vi "0-999 NUMBER TO STRING (SubVI).vi"(1 "A":dbl) -> (0 "element":string)   [LabVIEW 2019]
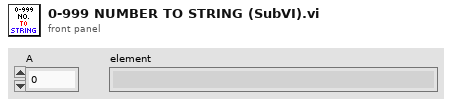
[diagram p1: front panel]
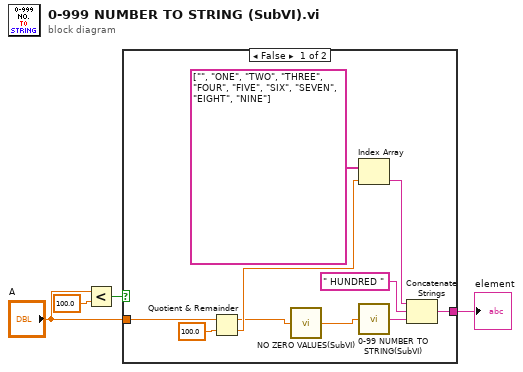
[diagram p0: block diagram]
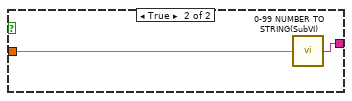
[diagram p2: hidden frame]
diagram:
  n1 = Less?(x="A", y=100.0) -> (x < y?=w1:bool)
  n2 = case shown="False" w1 {
    tunnel: "A" -> [w14 w16]
    tunnel: [w8 w15] -> w4
    frame False {
      n3 = Quotient & Remainder(x=w14, y=100.0) -> (x-y*floor(x/y)=w5:dbl, floor(x/y)=w12:dbl)
      n4 = call "NO ZERO VALUES(SubVI).vi"("Numeric"=w5) -> ("t"=w6:dbl)
      n5 = Index Array(array=string[] ["", "ONE", "TWO", "THREE", "FOUR", "FIVE", "SIX", "SEVEN", "EIGHT", "NINE"], index=w12) -> (element=w10:string)
      n6 = call "0-99 NUMBER TO STRING(SubVI).vi"("A"=w6) -> ("element"=w7:string)
      n7 = Concatenate Strings(w10, " HUNDRED " ("string"), w7) -> (w8:string)
    }
    frame True {
      n8 = call "0-99 NUMBER TO STRING(SubVI).vi"("A"=w16) -> ("element"=w15:string)
    }
  }
  "element" <- w4
